vi "GetDataSource.vi"(0 "appended path":path, 1 "ParametersCluster":T1={"Nl"=1.0, "subframe_type"=1.0, "cp_type"=0.0, "cfi"=1.0, "UL_subframe_num"=2.0, "prb_num"=100.0, "module_type"=enum."64QAM", "mimo_type"=1.0, "tbsize"=57336.0}) -> (4 "info_data":dbl[](array[numeric]), 6 "error IO":errorcluster)   [LabVIEW 2015]
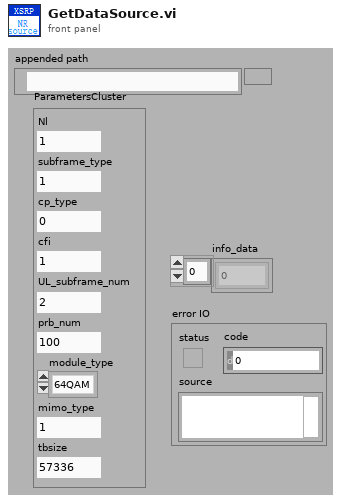
[diagram p1: front panel]
types:
  T1 = cluster{"Nl":dbl, "subframe_type":dbl, "cp_type":dbl, "cfi":dbl, "UL_subframe_num":dbl, "prb_num":dbl, "module_type":enum16{"", "QPSK", "16QAM", "64QAM"}, "mimo_type":dbl, "tbsize":dbl}
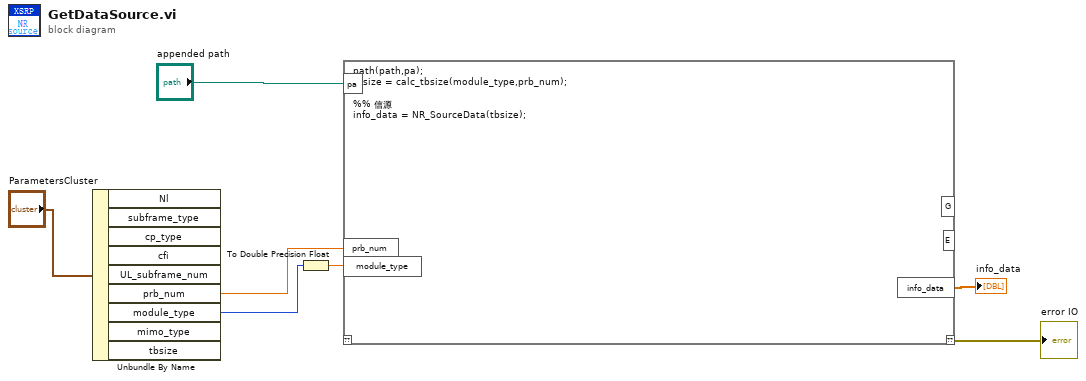
[diagram p0: block diagram]
diagram:
  n1 = Unbundle By Name("ParametersCluster") -> ("prb_num"=w3:dbl, "module_type"=w2:enum16{"", "QPSK", "16QAM", "64QAM"})  [unwired: 7 out]
  n2 = To Double Precision Float(number=w2) -> (double precision float=w1:dbl)
  n3 = script code="path(path,pa);\ntbsize = calc_tbsize(module_type,prb_num);\n\n%% 信源\ninfo_data = NR_SourceData(tbsize);"("pa"="appended path", "prb_num"=w3, "module_type"=w1) -> ("??"=→"error IO":errorcluster, "info_data"=→"info_data":dbl[])  [unwired: 3 out]
